vi "Write channel pointer.vi"(8 "error in (no error)":errorcluster, 10 "channel pointer":u64 format="%.0x", 11 "Runtime.Channel in":refnum<class "Runtime.Channel.lvclass">) -> (0 "error out":errorcluster, 3 "Runtime.Channel out":refnum<class "Runtime.Channel.lvclass">)   [LabVIEW 2016, in "Runtime.Channel.lvclass"]
uses:
  Runtime.Channel.lvclass
  Runtime.Channel.lvclass/Runtime.Channel.ctl
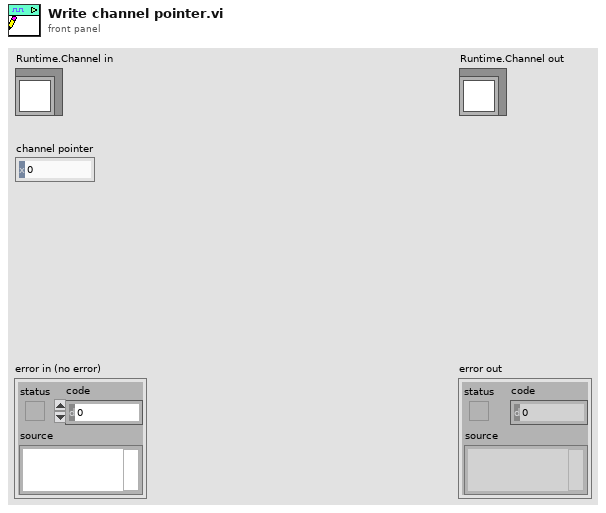
[diagram p1: front panel]
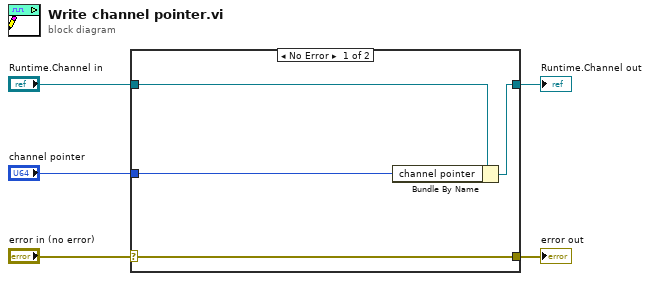
[diagram p0: block diagram]
diagram:
  n1 = case shown="No Error" "error in (no error)" {
    selector: "error in (no error)" -> [w9 w10]
    tunnel: [w9 w10] -> w4
    tunnel: [w7 w11] -> w2
    tunnel: "Runtime.Channel in" -> [w8 w11]
    tunnel: "channel pointer" -> [w6 _]
    frame No Error {
      n2 = Bundle By Name(cluster=w8, "channel pointer"=w6) -> (w7:refnum<class "Runtime.Channel.lvclass">)
    }
    frame Error {
    }
  }
  "error out" <- w4
  "Runtime.Channel out" <- w2
